vi "Write Data_Coils.vi"(8 "error in (no error)":errorcluster, 9 "register values":bool[](array[boolean]), 11 "Device in":refnum<class "RS232_Device.lvclass">) -> (0 "error out":errorcluster, 3 "Device out":refnum<class "RS232_Device.lvclass">)   [LabVIEW 2023, in "RS232_Device.lvclass"]
uses:
  RS232_Device.lvclass
  D:/SamparkProdLine/subVIs/DAQ Device/Modbus_Device/DAQ_Device.lvclass
  RS232_Device.lvclass/RS232_Device.ctl
panel:
  out "offset past match":i32
  out "resulting string":string
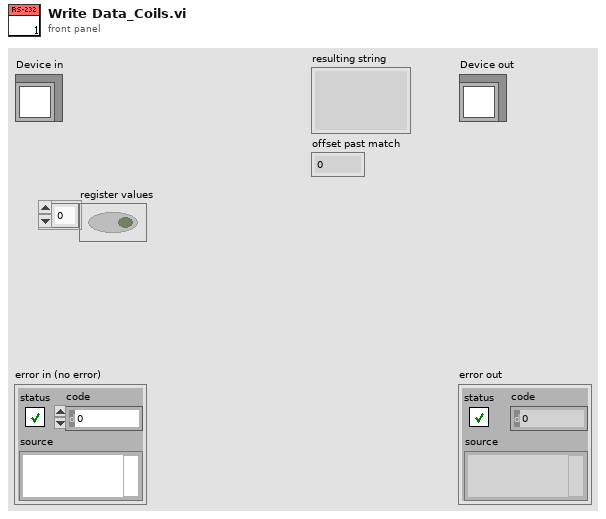
[diagram p1: front panel]
types:
  T1 = typedef "DAQ Device_IO ChannelsData.ctl" = cluster{"#DigitalInputs":u16, "StartAddress_DI":u16, "#DigitalOutputs":u16, "StartAddress_DO":u16, "#AnalogInputs":u16, "StartAddress_AI":u16, "#AnalogOutputs":u16, "StartAddress_AO":u16, "Coil_ReadData":bool[], "Coil_WriteData":bool[], "AI_Data":u16[], "AO_Data":u16[]}
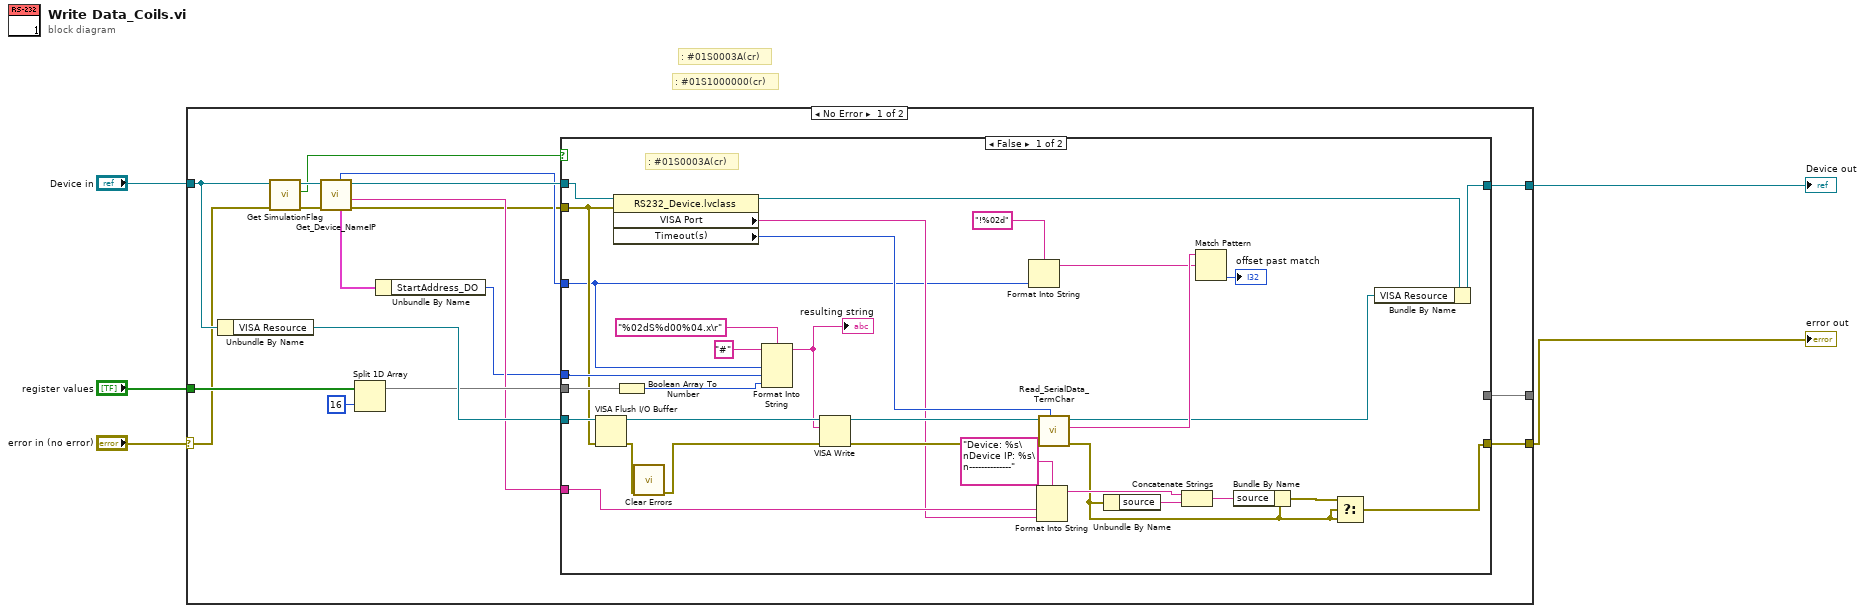
[diagram p0: block diagram]
diagram:
  # ": #01S1000000(cr)"
  # ": #01S0003A(cr)"
  n1 = case shown="No Error" "error in (no error)" {
    selector: "error in (no error)" -> [w8 w60]
    tunnel: [w22 w60] -> w2
    tunnel: [w23 w59] -> w3
    tunnel: "Device in" -> [w12 w59]
    tunnel: [w20 _] -> _
    tunnel: "register values" -> [w17 _]
    frame No Error {
      n2 = Unbundle By Name(w12) -> ("VISA Resource"=w21:refnum<visa-resource-name>)
      n3 = call-dynamic "Get SimulationFlag.vi"("error in (no error)"=w8, "Device in"=w12) -> ("error out"=w16:errorcluster, "Simulation?"=w9:bool, "Device out"=w13:refnum<class "RS232_Device.lvclass">)  [unwired: 7 in]
      n4 = call-dynamic "Get_Device_NameIP.vi"("error in (no error)"=w16, "Device in"=w13) -> ("error out"=w7:errorcluster, "Device Name"=w10:string, "Device out"=w14:refnum<class "RS232_Device.lvclass">, "IO Channels"=w15:T1, "Unit ID"=w11:u8)  [unwired: 4 in, 1 out]
      n5 = Split 1D Array(array=w17, index=16) -> (first subarray=w18:bool[])  [unwired: 1 out]
      n6 = Unbundle By Name(w15) -> ("StartAddress_DO"=w6:u16)
      n7 = case shown="False" w9 {
        tunnel: [w55 w58] -> w23
        tunnel: [w54 w56] -> w22
        tunnel: w21 -> [w53 _]
        tunnel: w14 -> [w30 w58]
        tunnel: w10 -> [w52 _]
        tunnel: [_ w57] -> w20
        tunnel: w18 -> [w33 w57]
        tunnel: w11 -> [w26 _]
        tunnel: w6 -> [w36 _]
        tunnel: w7 -> [w29 w56]
        frame False {
          # ": #01S0003A(cr)"
          n8 = VISA Flush I/O Buffer(VISA resource name=w53, error in (no error)=w29) -> (VISA resource name out=w46:refnum<visa-resource-name>, error out=w45:errorcluster)  [unwired: 1 in]
          n9 = property class="RS232_Device.lvclass"(reference=w30, error in=w29) -> (reference out=w31:refnum<class "RS232_Device.lvclass">, "VISA Port"=w27:string, "Timeout(s)"=w28:i32)  [unwired: 1 out]
          n10 = Boolean Array To Number(Boolean array=w33) -> (number=w34:u32)
          n11 = call <vilib>:"Clear Errors.vi"("error in (no error)"=w45) -> ("error out"=w44:errorcluster)  [unwired: 5 in, 1 out]
          n12 = Format Into String(format string="%02dS%d00%04.x\r", initial string="#", w26, w36, w34) -> (resulting string=w35:string)  [unwired: 1 in, 1 out]
          "resulting string" <- w35
          n13 = VISA Write(VISA resource name=w46, write buffer=w35, error in (no error)=w44) -> (VISA resource name out=w43:refnum<visa-resource-name>, error out=w42:errorcluster)  [unwired: 1 out]
          n14 = Format Into String(format string="!%02d" ("regular expression"), w26) -> (resulting string=w25:string)  [unwired: 2 in, 1 out]
          n15 = Format Into String(format string="Device: %s\nDevice IP: %s\n--------------", w52, w27) -> (resulting string=w48:string)  [unwired: 2 in, 1 out]
          n16 = call "Read_SerialData_TermChar.vi"("timeout (50ms)"=w28, "error in (no error)"=w42, "VISA Refnum in"=w43) -> ("error out"=w41:errorcluster, "StringData"=w40:string, "VISA Refnum out"=w39:refnum<visa-resource-name>)  [unwired: 6 in]
          n17 = Unbundle By Name(w41) -> ("source"=w50:string)
          n18 = Concatenate Strings(w48, w50) -> (w47:string)
          n19 = Match Pattern(string=w40, regular expression=w25) -> (offset past match=→"offset past match":i32)  [unwired: 1 in, 3 out]
          n20 = Bundle By Name(cluster=w41, "source"=w47) -> (w51:errorcluster)
          n21 = Select(t=w51, s=w41, f=w41) -> (s? t:f=w54:errorcluster)
          n22 = Bundle By Name(cluster=w31, "VISA Resource"=w39) -> (w55:refnum<class "RS232_Device.lvclass">)
        }
        frame True {
        }
      }
    }
    frame Error {
    }
  }
  "error out" <- w2
  "Device out" <- w3
